vi "AttrMapToJson.vi"(7 "Prototype":variant, 8 "error in (no error)":errorcluster, 11 "AttrMap":T1) -> (0 "error out":errorcluster, 3 "Json":string)   [LabVIEW 2019, in "lv-apt-json-file.lvlib"]
uses:
  lv-apt-json-file.lvlib
  Def-AttrMap.ctl
  <vilib>/addons/_JKI.lib/Serialization/JSON/JKI JSON Serialization.lvlib
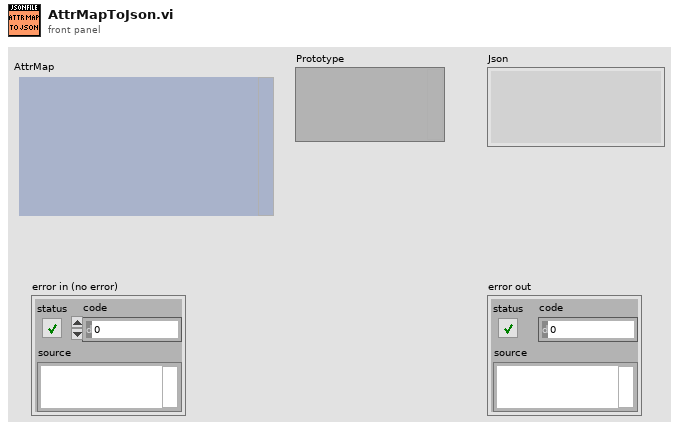
[diagram p1: front panel]
types:
  T1 = typedef "lv-apt-json-file.lvlib/Def-AttrMap.ctl" = variant
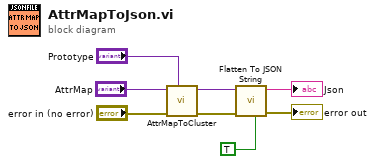
[diagram p0: block diagram]
diagram:
  n1 = call "AttrMapToCluster.vi"("Prototype"="Prototype", "error in (no error)"="error in (no error)", "AttrMap"="AttrMap") -> ("error out"=w2:errorcluster, "Cluster"=w3:variant)  [unwired: 7 in]
  n2 = call <vilib>:"Flatten To JSON String.vi"("Enums As String (F)"=TRUE, "error in (no error)"=w2, "Variant"=w3) -> ("error out"=→"error out":errorcluster, "JSON String"=→"Json":string)  [unwired: 7 in]
